vi "Login.vi"(8 "data out":string, 9 "Array Size":i32, 10 "Index Array":string[](array[string]), 11 "2D Arrays":string[][](array[string])) -> (1 "Enum":T1, 2 "String":string)   [LabVIEW 2023]
uses:
  Controller/ControllerATM.ctl
panel:
  # "Output"
  # "Input"
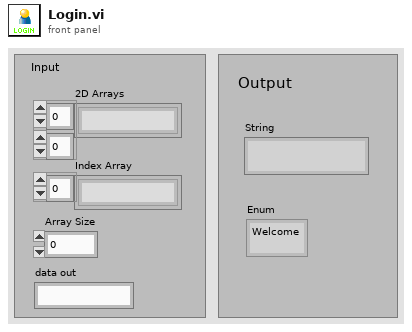
[diagram p1: front panel]
types:
  T1 = typedef "ControllerATM.ctl" = enum16{"Welcome", "Login", "Main", "Admin"}
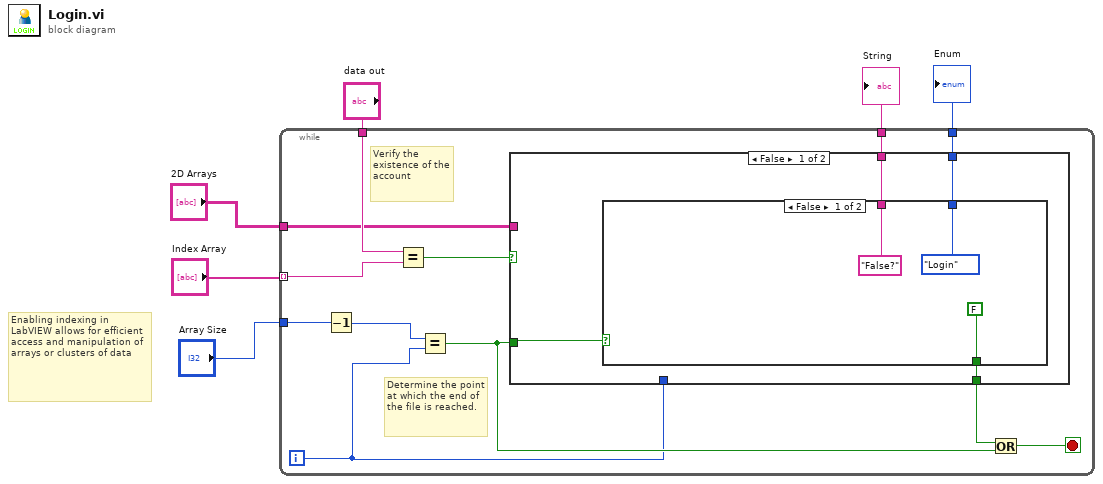
[diagram p0: block diagram]
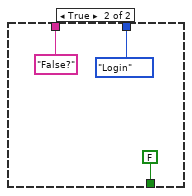
[diagram p2: hidden frame]
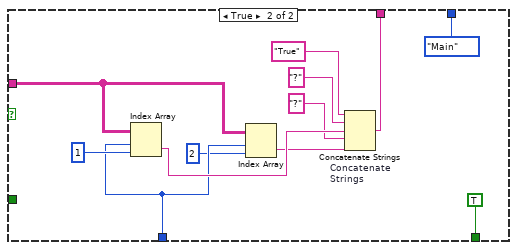
[diagram p3: hidden frame]
diagram:
  # "Enabling indexing in LabVIEW allows for efficient access and manipulation of arrays or clusters of data"
  n1 = while {
    tunnel: "data out" -> [w13]
    tunnel: "Index Array" -> [w12] mode=indexing
    tunnel: "2D Arrays" -> [w10]
    tunnel: "Array Size" -> [w18]
    tunnel: [w8] -> w2
    tunnel: [w7] -> w1
    i -> [w9]
    stop <- w15 stop-if-true
    # "Determine the point at which the end of the file is reached."
    # "Verify the existence of the account"
    n2 = Decrement(x=w18) -> (x-1=w17:i32)
    n3 = Equal?(x=w13, y=w12) -> (x = y?=w11:bool)
    n4 = Equal?(x=w17, y=w9) -> (x = y?=w14:bool)
    n5 = case shown="False" w11 {
      tunnel: w14 -> [w22 _]
      tunnel: [w20 TRUE] -> w16
      tunnel: w10 -> [_ w39]
      tunnel: w9 -> [_ w31]
      tunnel: [w21 w33] -> w8
      tunnel: [w19 ControllerATM."Main"] -> w7
      frame False {
        n6 = case shown="False" w22 {
          tunnel: ["False?" "False?"] -> w21
          tunnel: [ControllerATM."Login" ControllerATM."Login"] -> w19
          tunnel: [FALSE FALSE] -> w20
          frame False {
          }
          frame True {
          }
        }
      }
      frame True {
        n7 = Index Array "Index Array"(array=w39, index (row)=w31, index (col)=1 ("index (row)")) -> (element=w36:string)
        n8 = Index Array "Index Array"(array=w39, index (row)=w31, index (col)=2 ("index (row)")) -> (element=w34:string)
        n9 = Concatenate Strings "Concatenate\nStrings"("True" ("string"), "?" ("string"), w36, "?" ("string"), w34) -> (w33:string)
      }
    }
    n10 = Or(x=w16, y=w14) -> (x .or. y?=w15:bool)
  }
  "String" <- w2
  "Enum" <- w1
